vi "dezimal zeichen.vi"() -> ()   [LabVIEW 2010, in "Licor-Steuerung.lvlib"]
uses:
  Licor-Steuerung.lvlib
panel:
  in  "String":string
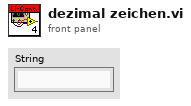
[diagram p1: front panel]
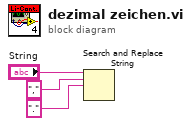
[diagram p0: block diagram]
diagram:
  n1 = Search and Replace String(input string="String", search string="," ("Such-String"), replace string="." ("Ersetzungs-String (\"\")")) -> ()  [unwired: 5 in, 4 out]
